vi "New.vi"(8 "error in (no error)":errorcluster, 10 "object":refnum<class "_ISerializable.lvclass">) -> (0 "error out":errorcluster, 3 "Serializer out":refnum<class "Serializer.lvclass">)   [LabVIEW 2018, in "Serializer.lvclass"]
uses:
  Serializer.lvclass
  _Serializable Base Object/_ISerializable.lvclass
  Serializer.lvclass/Serializer.ctl
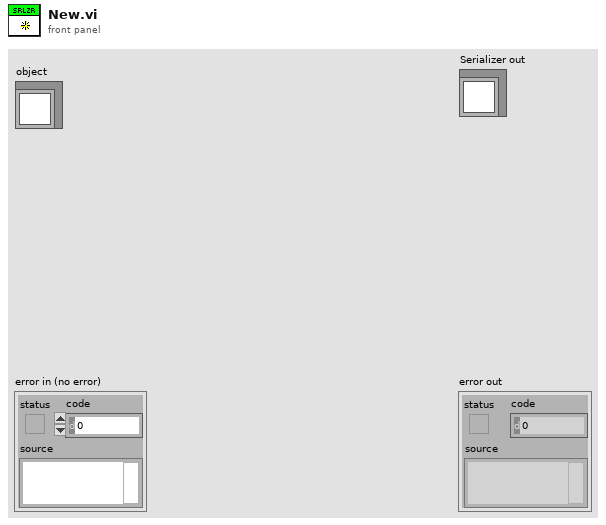
[diagram p1: front panel]
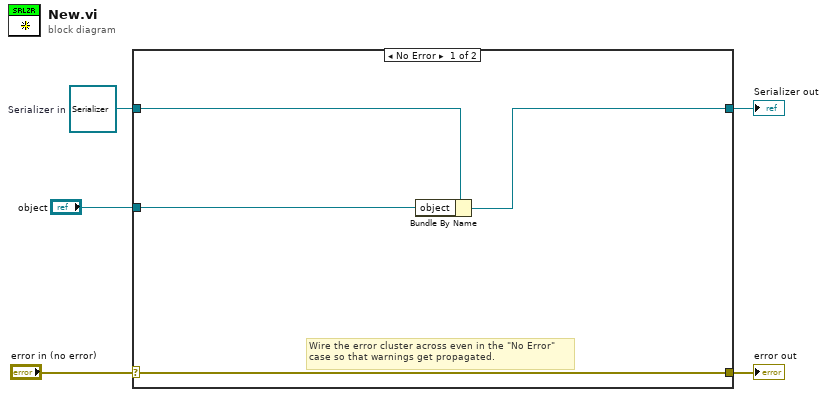
[diagram p0: block diagram]
diagram:
  w3 = refnum<class "Serializer.lvclass"> refnum  # Serializer in
  n1 = case shown="No Error" "error in (no error)" {
    selector: "error in (no error)" -> [w9 w11]
    tunnel: [w9 w11] -> w4
    tunnel: [w8 w10] -> w2
    tunnel: w3 -> [w7 w10]
    tunnel: "object" -> [w6 _]
    frame No Error {
      # "Wire the error cluster across even in the \"No Error\"\ncase so that warnings get propagated."
      n2 = Bundle By Name(cluster=w7, "object"=w6) -> (w8:refnum<class "Serializer.lvclass">)
    }
    frame Error {
    }
  }
  "error out" <- w4
  "Serializer out" <- w2
